vi "Set To Array.vi"(11 "Set":set{string}(c389)) -> (3 "Array[]":string[](array[string]))   [LabVIEW 2019, in "SLL Environment Variable.lvlib"]
doc: "Convert set to array"
uses:
  SLL Environment Variable.lvlib
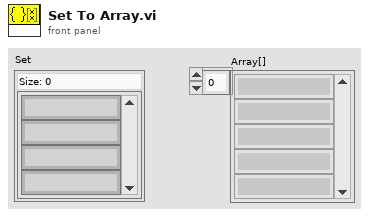
[diagram p1: front panel]
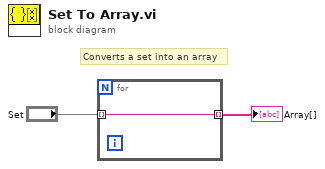
[diagram p0: block diagram]
diagram:
  # "Converts a set into an array"
  n1 = for {
    tunnel: [w3] -> w2 mode=indexing
    tunnel: "Set" -> [w3] mode=indexing
  }
  "Array[]" <- w2
